vi "1_4.vi"() -> ()   [LabVIEW 2020]
panel:
  out "Out":dbl
  in  "In":dbl
  in  "Select":bool caption="Boolean"
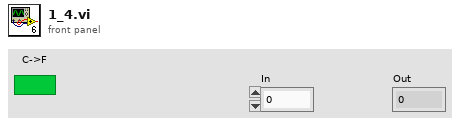
[diagram p1: front panel]
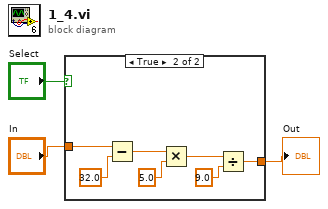
[diagram p0: block diagram]
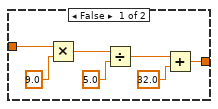
[diagram p2: hidden frame]
diagram:
  n1 = case shown="True" "Select" {
    tunnel: "In" -> [w7 w16]
    tunnel: [w4 w11] -> w1
    frame False {
      n2 = Multiply(x=w7, y=9.0) -> (x*y=w6:dbl)
      n3 = Divide(x=w6, y=5.0) -> (x/y=w5:dbl)
      n4 = Add(x=w5, y=32.0) -> (x+y=w4:dbl)
    }
    frame True {
      n5 = Subtract(x=w16, y=32.0) -> (x-y=w14:dbl)
      n6 = Multiply(x=w14, y=5.0) -> (x*y=w12:dbl)
      n7 = Divide(x=w12, y=9.0) -> (x/y=w11:dbl)
    }
  }
  "Out" <- w1
